vi "lecture1-b.vi"() -> ()   [LabVIEW 2014]
panel:
  out "A - B":dbl format="%#_13g"
  out "A + B":dbl format="%#_13g"
  in  "B":dbl format="%#_13g"
  in  "A":dbl format="%#_13g"
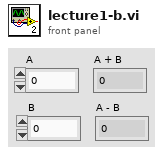
[diagram p1: front panel]
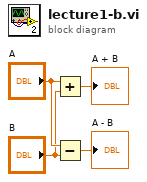
[diagram p0: block diagram]
diagram:
  n1 = Add(x="A", y="B") -> (x+y=→"A + B":dbl)
  n2 = Subtract(x="A", y="B") -> (x-y=→"A - B":dbl)
